vi "bulk Write Tx Only.vi"(9 "param_length":u16, 10 "protocol_version":i32, 11 "port_num":i32) -> ()   [LabVIEW 2015, in "dxl_x86_c.lvlib"]
doc: "WINDECLSPEC void bulkWriteTxOnly (int port_num, int protocol_version, uint16_t param_length);"
uses:
  dxl_x86_c.lvlib
  dxl_x86_c.dll
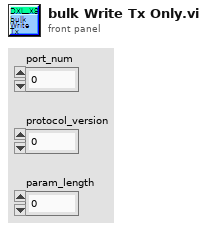
[diagram p1: front panel]
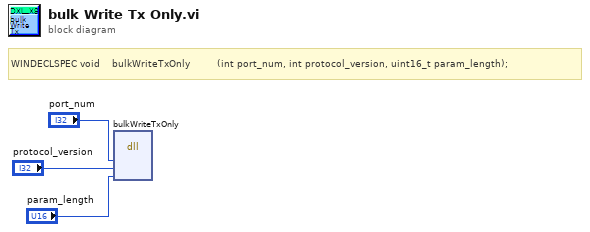
[diagram p0: block diagram]
diagram:
  # "WINDECLSPEC void    bulkWriteTxOnly         (int port_num, int protocol_version, uint16_t param_length);"
  n1 = dll-call lib="C:/Users/Platform/Desktop/LabVIEW/dxl_x86_c.lvlib/dxl_x86_c.*" fn="bulkWriteTxOnly"("port_num"="port_num", "protocol_version"="protocol_version", "param_length"="param_length") -> ()  [unwired: 7 in, 2 out]
